vi "OpenByRefnum.vi"(0 "VI refnum":refnum<vi>, 1 "Application reference":refnum<vi> caption="Application reference (Local)", 9 "Reentrancy mode":T2=enum."Auto" caption="Reentrancy mode (Auto)", 11 "Error in":errorcluster caption="Error in (no error)") -> (4 "VI refnum out":refnum<vi>, 6 "VI refnum opened?":bool, 8 "Last execution state":T1(ring), 10 "VI refnum opened as reentrant?":bool, 15 "Error out":errorcluster)   [LabVIEW 2017, in "VILauncher.lvlib"]
doc: "Opens a reference to a dynamic VI specified by <B>VI refnum</B> and returns the reference to the opened VI in <B>VI refnum out</B>. Remember to close the VI reference when you're done using it.\n\nThe optional <B>Application reference</B> can be used to specify another application instance to open the VI reference in. Use the Open Application Reference LabVIEW function to open another application reference.\n\nUse the optional <B>Reentrancy mode</B> input to specify whether the dynamic VI should be opened as a reentrant or a non-reentrant instance. Set this to Auto (default) to first try as reentrant, and if that fails, as non-reentrant. The <B>VI refnum opened as reentrant?</B> output will reflect the instantiation mode.\n\nThe <B>VI refnum opened?</B> output will only be True if the dynamic VI's <B>Last execution state</B> is \"Idle\" or \"Running\".\n\nThis VI is reentrant, and it doesn't run if there is an error on <B>Error in</B>.\n\nSteen Schmidt\nGPower\n26/12 2012"
uses:
  VILauncher.lvlib
  Error/GPError.lvlib
  Typedefs/ReentrancyMode.ctl
panel:
  # "Copyright © 2013\nGPower\nSee enclosed license file for terms and conditions"
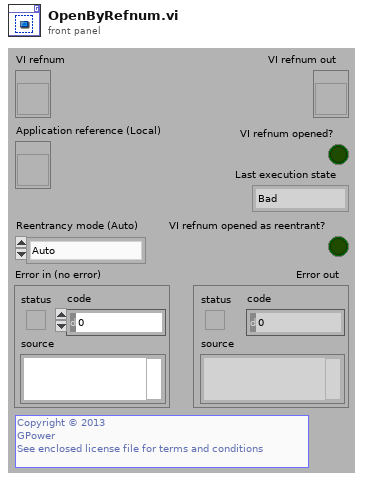
[diagram p1: front panel]
types:
  T1 = enum32{"Bad", "Idle", "Run top level", "Running"}
  T2 = typedef "VILauncher.lvlib/ReentrancyMode.ctl" = enum16{"Reentrant", "Non-reentrant", "Auto"}
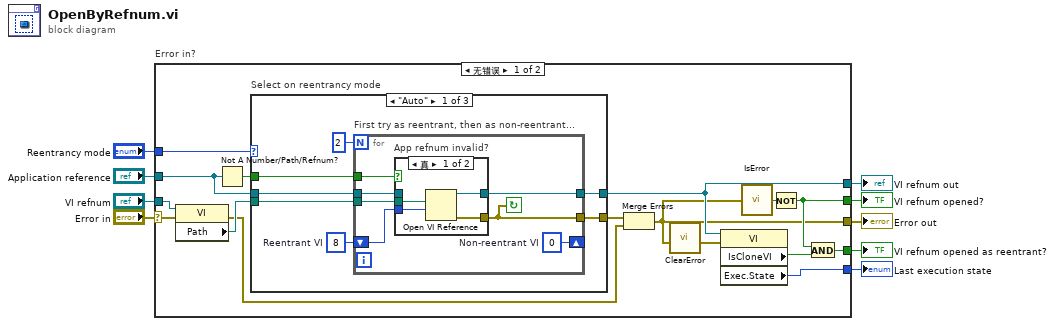
[diagram p0: block diagram]
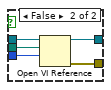
[diagram p2: hidden frame]
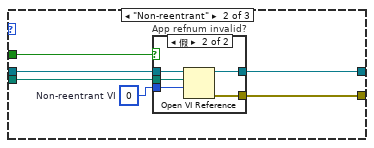
[diagram p3: hidden frame]
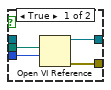
[diagram p4: hidden frame]
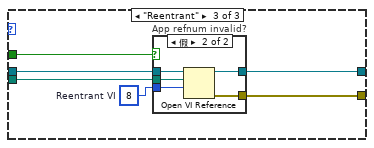
[diagram p5: hidden frame]
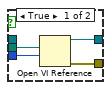
[diagram p6: hidden frame]
diagram:
  n1 = case "Error in?" shown="无错误" "Error in" {
    selector: "Error in" -> [w22 w79]
    tunnel: [w10 w79] -> w8
    tunnel: "Application reference" -> [w24 _]
    tunnel: "Reentrancy mode" -> [w25 _]
    tunnel: [w11 _] -> w5
    tunnel: [w13 _] -> w4
    tunnel: [w12 _] -> w1
    tunnel: [w14 _] -> w3
    tunnel: "VI refnum" -> [w20 _]
    frame No Error {
      n2 = property class="VI"(reference=w20, error in=w22) -> (error out=w18:errorcluster, "Path"=w21:path)  [unwired: 1 out]
      n3 = Not A Number/Path/Refnum?(number/path/refnum=w24) -> (NaN/Path/Refnum?=w23:bool)
      n4 = case "Select on reentrancy mode" shown="\"Auto\"" w25 {
        tunnel: w21 -> [w30 w50 w65]
        tunnel: w24 -> [w29 w51 w66]
        tunnel: [w28 w53 w68] -> w14
        tunnel: [w27 w54 w69] -> w19
        tunnel: w23 -> [w26 w52 w67]
        frame "Auto" {
          w32 = 8  # Reentrant VI
          n5 = for "First try as reentrant, then as non-reentrant..." {
            N: 2 -> [_]
            shift-right: [w38] -> _
            shift-left: w32 -> [w39]
            tunnel: w30 -> [w37]
            tunnel: w29 -> [w36]
            tunnel: [w35] -> w28
            tunnel: [w34] -> w27
            tunnel: w26 -> [w33]
            stop <- w34 continue-if-true
            w38 = 0  # Non-reentrant VI
            n6 = case "App refnum invalid?" shown="真" w33 {
              tunnel: w39 -> [w43 w48]
              tunnel: w37 -> [w42 w47]
              tunnel: w36 -> [_ w46]
              tunnel: [w41 w45] -> w35
              tunnel: [w40 w44] -> w34
              frame True {
                n7 = Open VI Reference(vi path=w42, options=w43) -> (vi reference=w41:refnum<vi>, error out=w40:errorcluster)  [unwired: 2 in, 2 out]
              }
              frame False {
                n8 = Open VI Reference(application reference (local)=w46, vi path=w47, options=w48) -> (vi reference=w45:refnum<vi>, error out=w44:errorcluster)  [unwired: 2 in, 1 out]
              }
            }
          }
        }
        frame "Non-reentrant" {
          w49 = 0  # Non-reentrant VI
          n9 = case "App refnum invalid?" shown="假" w52 {
            tunnel: w49 -> [w58 w63]
            tunnel: w50 -> [w57 w62]
            tunnel: w51 -> [_ w61]
            tunnel: [w56 w60] -> w53
            tunnel: [w55 w59] -> w54
            frame True {
              n10 = Open VI Reference(vi path=w57, options=w58) -> (vi reference=w56:refnum<vi>, error out=w55:errorcluster)  [unwired: 2 in, 2 out]
            }
            frame False {
              n11 = Open VI Reference(application reference (local)=w61, vi path=w62, options=w63) -> (vi reference=w60:refnum<vi>, error out=w59:errorcluster)  [unwired: 2 in, 1 out]
            }
          }
        }
        frame "Reentrant" {
          w64 = 8  # Reentrant VI
          n12 = case "App refnum invalid?" shown="假" w67 {
            tunnel: w64 -> [w73 w78]
            tunnel: w65 -> [w72 w77]
            tunnel: w66 -> [_ w76]
            tunnel: [w71 w75] -> w68
            tunnel: [w70 w74] -> w69
            frame True {
              n13 = Open VI Reference(vi path=w72, options=w73) -> (vi reference=w71:refnum<vi>, error out=w70:errorcluster)  [unwired: 2 in, 2 out]
            }
            frame False {
              n14 = Open VI Reference(application reference (local)=w76, vi path=w77, options=w78) -> (vi reference=w75:refnum<vi>, error out=w74:errorcluster)  [unwired: 2 in, 1 out]
            }
          }
        }
      }
      n15 = Merge Errors(w19, w18) -> (w10:errorcluster)
      n16 = call "ClearError.vi"("Error in"=w10) -> ("Error out"=w17:errorcluster)  [unwired: 10 in]
      n17 = property class="VI"(reference=w14, error in=w17) -> ("IsCloneVI"=w15:bool, "Exec.State"=w12:T1)  [unwired: 2 out]
      n18 = call "IsError.vi"("Error in"=w10) -> ("Error?"=w16:bool)  [unwired: 4 in]
      n19 = Not(x=w16) -> (.not. x?=w11:bool)
      n20 = And(x=w11, y=w15) -> (x .and. y?=w13:bool)
    }
    frame Error {
    }
  }
  "Error out" <- w8
  "VI refnum out" <- w3
  "Last execution state" <- w1
  "VI refnum opened as reentrant?" <- w4
  "VI refnum opened?" <- w5
